vi "setPressedButtonRef.vi"(8 "error in (no error)":errorcluster, 10 "Pressed Button Ref":refnum<vi>, 11 "Check Move in":refnum<class "Check Move.lvclass">) -> (0 "error out":errorcluster, 3 "Check Move out":refnum<class "Check Move.lvclass">)   [LabVIEW 2019, in "Check Move.lvclass"]
uses:
  Check Move.lvclass
  Check Move.lvclass/Check Move.ctl
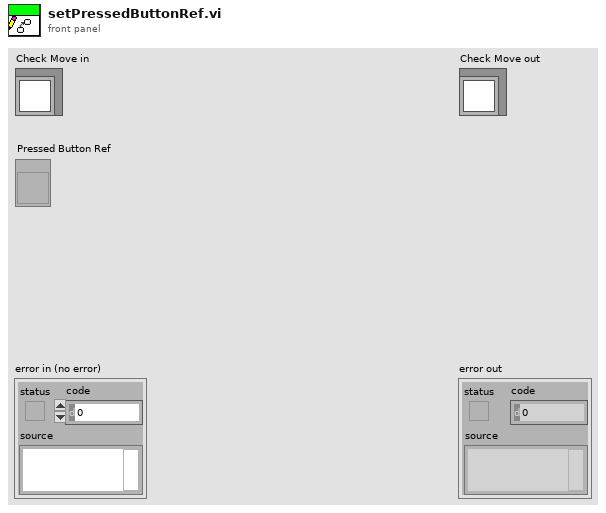
[diagram p1: front panel]
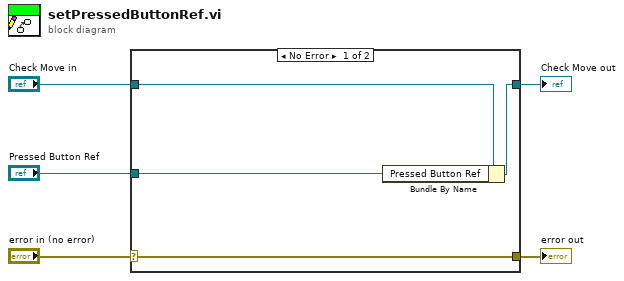
[diagram p0: block diagram]
diagram:
  n1 = case shown="No Error" "error in (no error)" {
    selector: "error in (no error)" -> [w9 w10]
    tunnel: [w9 w10] -> w4
    tunnel: [w7 w11] -> w2
    tunnel: "Check Move in" -> [w8 w11]
    tunnel: "Pressed Button Ref" -> [w6 _]
    frame No Error {
      n2 = Bundle By Name(cluster=w8, "Pressed Button Ref"=w6) -> (w7:refnum<class "Check Move.lvclass">)
    }
    frame Error {
    }
  }
  "error out" <- w4
  "Check Move out" <- w2
